vi "Deploy.vi"(8 "error in (no error)":errorcluster, 9 "Deploy?":bool, 11 "Hatch Concrete in":refnum<class "Hatch Concrete.lvclass">) -> (0 "error out":errorcluster, 3 "Hatch Concrete out":refnum<class "Hatch Concrete.lvclass">)   [LabVIEW 2018, in "Hatch.lvlib" / "Hatch Concrete.lvclass"]
uses:
  Hatch Concrete.lvclass
  Hatch Concrete.lvclass/Hatch Concrete.ctl
  <vilib>/Rock Robotics/WPI/Solenoid/WPI_SolenoidValue.ctl
  <vilib>/Rock Robotics/WPI/Solenoid/WPI_SolenoidSetEnum.vi
  Hatch.lvclass
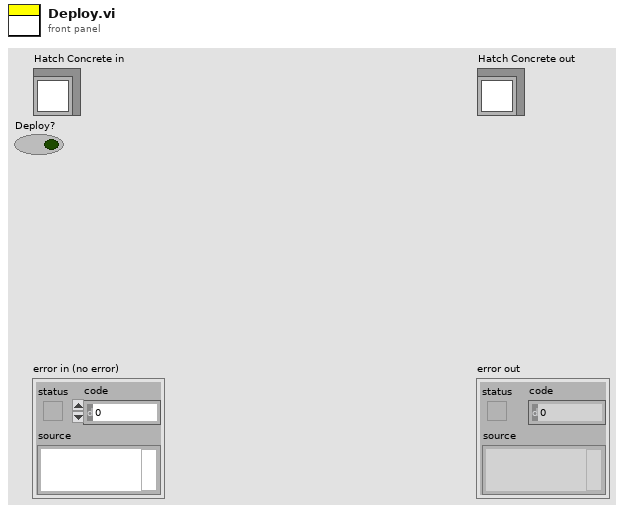
[diagram p1: front panel]
types:
  T1 = typedef "WPI_SolenoidValue.ctl" = enum16{"Off", "On", "Forward", "Reverse"}
  T2 = typedef "WPI_SolenoidDevRef.ctl" = cluster{"DevStatus":errorcluster, "Pneumatics Control Module":u8, "Forward Solenoid Channel":T3, "Reverse Solenoid Channel":T3}
  T3 = typedef "WPI_SolenoidChannel.ctl" = enum8{"Solenoid 0", "Solenoid 1", "Solenoid 2", "Solenoid 3", "Solenoid 4", "Solenoid 5", "Solenoid 6", "Solenoid 7", "Invalid"}
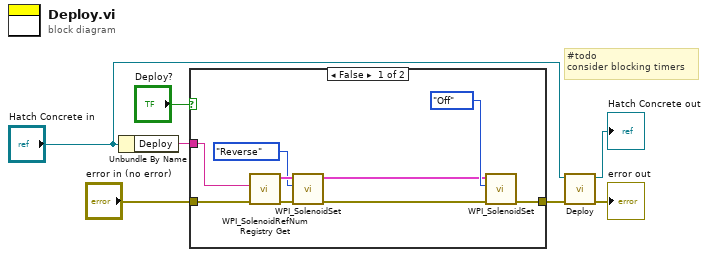
[diagram p0: block diagram]
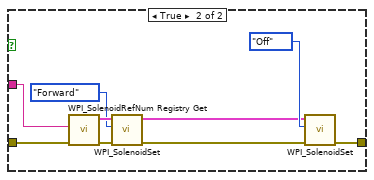
[diagram p2: hidden frame]
diagram:
  # "#todo\nconsider blocking timers"
  n1 = Unbundle By Name("Hatch Concrete in") -> ("Deploy"=w4:string)
  n2 = case shown="False" "Deploy?" {
    tunnel: w4 -> [w13 w22]
    tunnel: "error in (no error)" -> [w12 w20]
    tunnel: [w11 w21] -> w1
    frame False {
      n3 = call <vilib>:"WPI_SolenoidRefNum Registry Get.vi"("error in (no error)"=w12, "refnum name"=w13) -> ("error out"=w15:errorcluster, "SolenoidDevRef"=w16:T2)  [unwired: 8 in]
      n4 = call-poly <vilib>:"WPI_SolenoidSet.vi"("error in (no error)"=w15, "Value"=WPI_SolenoidValue."Reverse", "SolenoidDevRef"=w16) -> ("error out"=w8:errorcluster, "SolenoidDevRef"=w9:T2)  [unwired: 7 in]
      n5 = call-poly <vilib>:"WPI_SolenoidSet.vi"("error in (no error)"=w8, "Value"=WPI_SolenoidValue."Off", "SolenoidDevRef"=w9) -> ("error out"=w11:errorcluster)  [unwired: 7 in, 1 out]
    }
    frame True {
      n6 = call <vilib>:"WPI_SolenoidRefNum Registry Get.vi"("error in (no error)"=w20, "refnum name"=w22) -> ("error out"=w25:errorcluster, "SolenoidDevRef"=w24:T2)  [unwired: 8 in]
      n7 = call-poly <vilib>:"WPI_SolenoidSet.vi"("error in (no error)"=w25, "Value"=WPI_SolenoidValue."Forward", "SolenoidDevRef"=w24) -> ("error out"=w17:errorcluster, "SolenoidDevRef"=w18:T2)  [unwired: 7 in]
      n8 = call-poly <vilib>:"WPI_SolenoidSet.vi"("error in (no error)"=w17, "Value"=WPI_SolenoidValue."Off", "SolenoidDevRef"=w18) -> ("error out"=w21:errorcluster)  [unwired: 7 in, 1 out]
    }
  }
  n9 = call-parent "Deploy.vi"("error in (no error)"=w1, "Hatch in"="Hatch Concrete in") -> ("error out"=→"error out":errorcluster, "Hatch out"=→"Hatch Concrete out":refnum<class "Hatch Concrete.lvclass">)  [unwired: 8 in]
